vi "Chart_to_GraphXY.vi"(5 "Time window":u16=20, 6 "reference in":cluster{"Tempi":dbl[], "Valori":dbl[]}[](array[cluster])=[{"Tempi"=[], "Valori"=[]}], 7 "Function":T1, 8 "error in":errorcluster, 9 "Index plot":u8, 10 "Valore in":dbl=30.0, 11 "Tempo in":dbl) -> (0 "error out":errorcluster, 1 "Valori out":dbl[](array[numeric]), 2 "Tempo out":dbl[](array[numeric]), 3 "XY Graph":cluster{"Tempi":dbl[], "Valori":dbl[]}[](graph), 4 "reference out":cluster{"Tempi":dbl[], "Valori":dbl[]}[](array[cluster]))   [LabVIEW 2015, in "My Graphs.lvlib"]
uses:
  My Graphs.lvlib
  Chart to Graph enum.ctl
  <vilib>/Utility/error.llb/Error Cluster From Error Code.vi
  <vilib>/ErrorRing/Error Ring.xnode
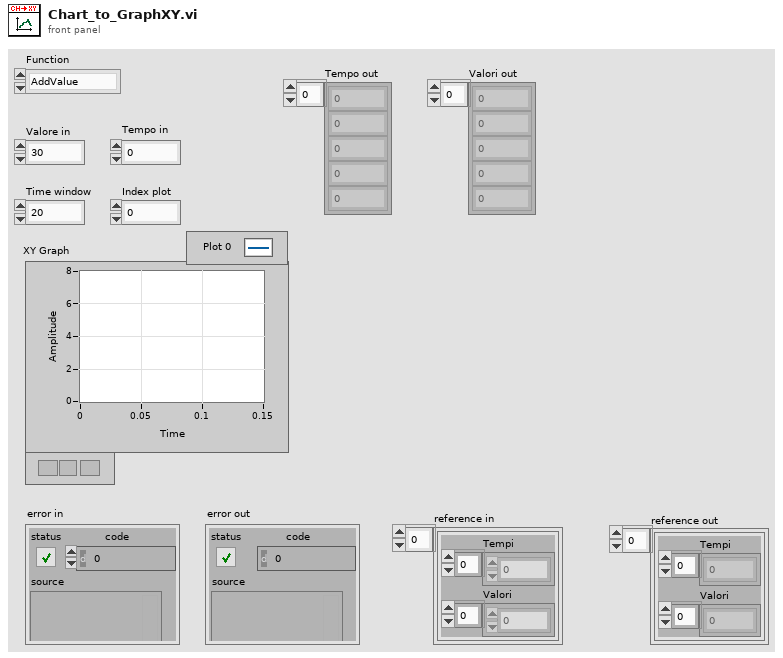
[diagram p1: front panel]
types:
  T1 = typedef "My Graphs.lvlib/Chart to Graph enum.ctl" = enum16{"AddValue", "Reset", "Delete_old"}
  T2 = cluster{"status":bool, "code":bool, "source":bool}
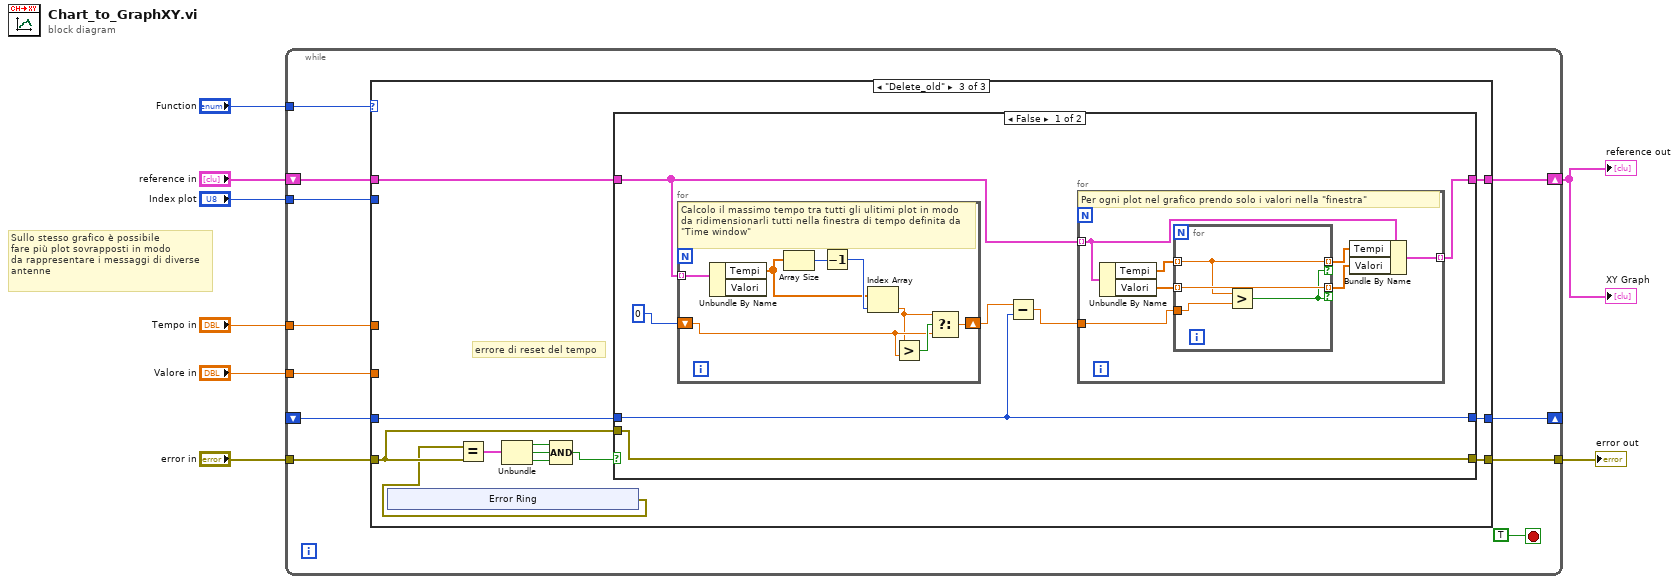
[diagram p0: block diagram]
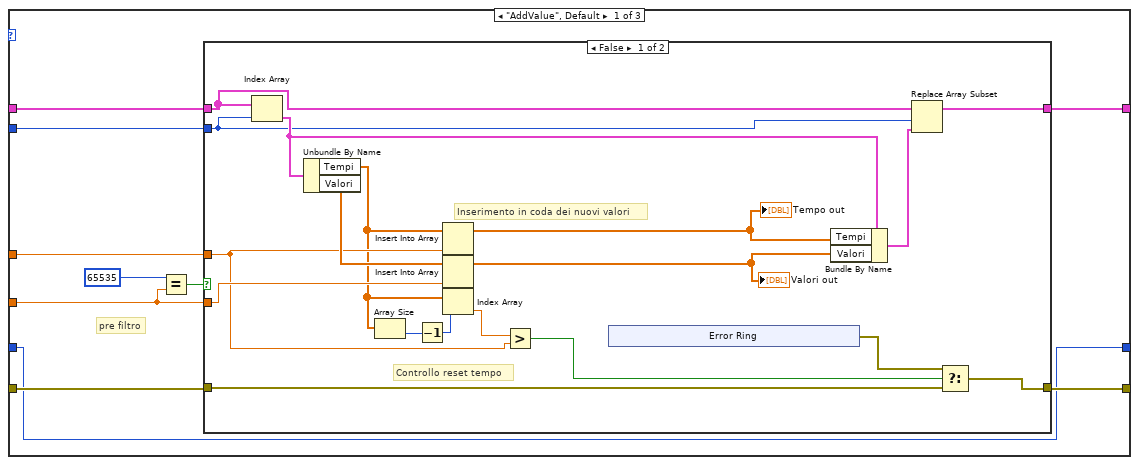
[diagram p2: hidden frame]
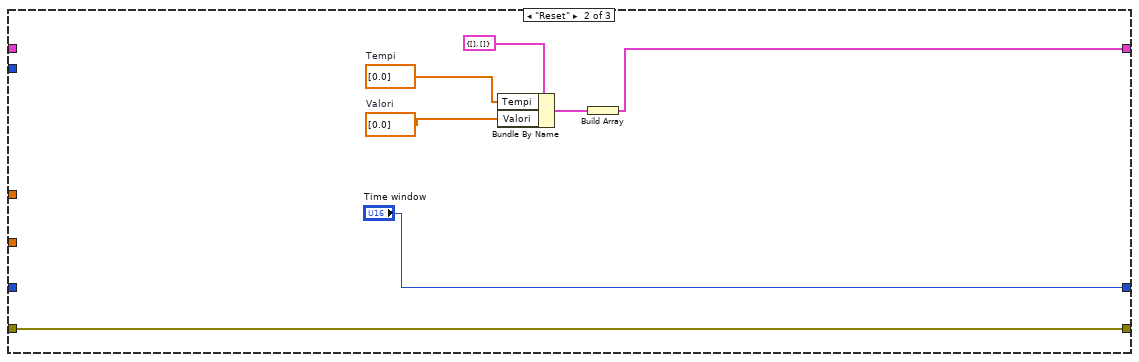
[diagram p4: hidden frame]
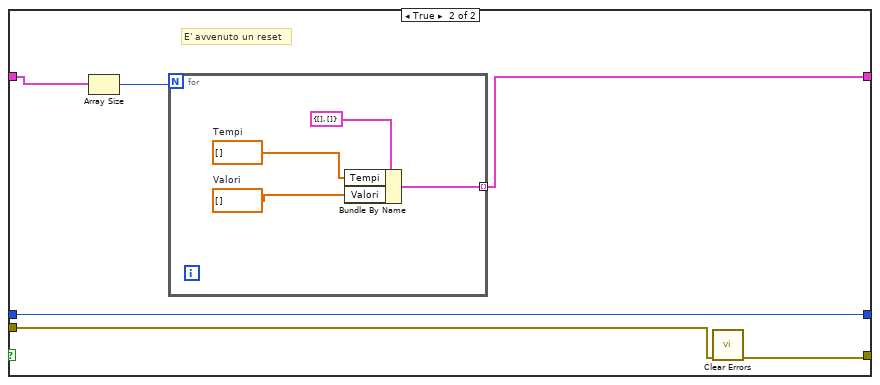
[diagram p5: hidden frame]
diagram:
  # "Sullo stesso grafico è possibile\nfare più plot sovrapposti in modo\nda rappresentare i messaggi di diverse\nantenne"
  n1 = while {
    tunnel: "Function" -> [w18]
    tunnel: "Tempo in" -> [w15]
    tunnel: "Valore in" -> [w12]
    tunnel: "error in" -> [w14]
    tunnel: [w13] -> w4
    tunnel: "Index plot" -> [w11]
    shift-right: [w17] -> w2
    shift-left: "reference in" -> [w16]
    shift-right: [w9] -> _
    shift-left: _ -> [w10]
    stop <- TRUE stop-if-true
    n2 = case shown="\"Delete_old\"" w18 {
      tunnel: w16 -> [w27 _ w73]
      tunnel: w15 -> [w29 _ _]
      tunnel: w12 -> [w25 _ _]
      tunnel: w14 -> [w24 w59 w64]
      tunnel: [w23 w59 w65] -> w13
      tunnel: [w26 w57 w71] -> w17
      tunnel: w11 -> [w28 _ _]
      tunnel: w10 -> [w20 _ w72]
      tunnel: [w20 "Time window" w63] -> w9
      frame "AddValue", Default {
        # "pre filtro"
        n3 = Equal?(x=65535, y=w25) -> (x = y?=w22:bool)
        n4 = case shown="False" w22 {
          tunnel: w29 -> [w40 _]
          tunnel: w28 -> [w33 _]
          tunnel: w27 -> [w35 w53]
          tunnel: [w45 w53] -> w26
          tunnel: w25 -> [w46 _]
          tunnel: w24 -> [w38 w54]
          tunnel: [w36 w54] -> w23
          frame False {
            # "Inserimento in coda dei nuovi valori"
            # "Controllo reset tempo"
            n5 = Index Array(array=w35, index=w33) -> (element=w34:cluster{"Tempi":dbl[], "Valori":dbl[]})
            n6 = Unbundle By Name(w34) -> ("Tempi"=w39:dbl[], "Valori"=w42:dbl[])
            n7 = Array Size(array=w39) -> (size(s)=w43:i32)
            n8 = Decrement(x=w43) -> (x-1=w44:i32)
            n9 = Insert Into Array(array=w39, new element=w40) -> (w31:dbl[])  [unwired: 1 in]
            "Tempo out" <- w31
            n10 = Insert Into Array(array=w42, new element=w46) -> (w30:dbl[])  [unwired: 1 in]
            "Valori out" <- w30
            n11 = Index Array(array=w39, index=w44) -> (element=w41:dbl)
            n12 = Greater?(x=w41, y=w40) -> (0:w37:bool)
            n13 = xnode "Error Ring"() -> ("error out"=w32:errorcluster)
            n14 = Bundle By Name(cluster=w34, "Tempi"=w31, "Valori"=w30) -> (w47:cluster{"Tempi":dbl[], "Valori":dbl[]})
            n15 = Replace Array Subset(array=w35, new element=w47, index=w33) -> (w45:cluster{"Tempi":dbl[], "Valori":dbl[]}[])
            n16 = Select(t=w32, s=w37, f=w38) -> (s? t:f=w36:errorcluster)
          }
          frame True {
          }
        }
      }
      frame "Reset" {
        w60 = dbl[] [0.0]  # Valori
        w61 = dbl[] [0.0]  # Tempi
        n17 = Bundle By Name(cluster=cluster{"Tempi":dbl[], "Valori":dbl[]} {"Tempi"=[], "Valori"=[]} ("input cluster"), "Tempi"=w61, "Valori"=w60) -> (w56:cluster{"Tempi":dbl[], "Valori":dbl[]})
        n18 = Build Array(w56) -> (w57:cluster{"Tempi":dbl[], "Valori":dbl[]}[])
      }
      frame "Delete_old" {
        # "errore di reset del tempo"
        n19 = xnode "Error Ring"() -> ("error out"=w62:errorcluster)
        n20 = Equal?(x=w62, y=w64) -> (x = y?=w70:T2)
        n21 = Unbundle(w70) -> ("status"=w69:bool, "code"=w68:bool, "source"=w67:bool)
        n22 = Compound Arithmetic op=AND(w69, w68, w67) -> (w66:bool)
        n23 = case shown="False" w66 {
          tunnel: w73 -> [w84 w109]
          tunnel: w72 -> [w79 w105]
          tunnel: [w81 w108] -> w71
          tunnel: [w80 w107] -> w65
          tunnel: w64 -> [w80 w106]
          tunnel: [w79 w105] -> w63
          frame False {
            n24 = for {
              tunnel: w84 -> [w104] mode=indexing
              shift-right: [w100] -> w83
              shift-left: 0 -> [w98]
              # "Calcolo il massimo tempo tra tutti gli ulitimi plot in modo da ridimensionarli tutti nella finestra di tempo definita da \"Time window\""
              n25 = Unbundle By Name(w104) -> ("Tempi"=w101:dbl[])  [unwired: 1 out]
              n26 = Array Size(array=w101) -> (size(s)=w103:i32)
              n27 = Decrement(x=w103) -> (x-1=w102:i32)
              n28 = Index Array(array=w101, index=w102) -> (element=w97:dbl)
              n29 = Greater?(x=w97, y=w98) -> (0:w99:bool)
              n30 = Select(t=w97, s=w99, f=w98) -> (s? t:f=w100:dbl)
            }
            n31 = Subtract(x=w83, y=w79) -> (x-y=w82:dbl)
            n32 = for {
              tunnel: w84 -> [w89] mode=indexing
              tunnel: w82 -> [w90]
              tunnel: [w86] -> w81 mode=indexing
              # "Per ogni plot nel grafico prendo solo i valori nella \"finestra\""
              n33 = Unbundle By Name(w89) -> ("Tempi"=w92:dbl[], "Valori"=w91:dbl[])
              n34 = for {
                tunnel: w92 -> [w94] mode=indexing
                tunnel: w91 -> [w96] mode=indexing
                tunnel: w90 -> [w95]
                tunnel: [w94] -> w88 mode=indexing if=w93
                tunnel: [w96] -> w87 mode=indexing if=w93
                n35 = Greater?(x=w94, y=w95) -> (0:w93:bool)
              }
              n36 = Bundle By Name(cluster=w89, "Tempi"=w88, "Valori"=w87) -> (w86:cluster{"Tempi":dbl[], "Valori":dbl[]})
            }
          }
          frame True {
            # "E' avvenuto un reset"
            n37 = Array Size(array=w109) -> (size(s)=w110:i32)
            n38 = for {
              N: w110 -> [_]
              tunnel: [w111] -> w108 mode=indexing
              w113 = dbl[] []  # Valori
              w114 = dbl[] []  # Tempi
              n39 = Bundle By Name(cluster=cluster{"Tempi":dbl[], "Valori":dbl[]} {"Tempi"=[], "Valori"=[]} ("input cluster"), "Tempi"=w114, "Valori"=w113) -> (w111:cluster{"Tempi":dbl[], "Valori":dbl[]})
            }
            n40 = call <vilib>:"Clear Errors.vi"("error in (no error)"=w106) -> ("error out"=w107:errorcluster)  [unwired: 5 in, 1 out]
          }
        }
      }
    }
  }
  "XY Graph" <- w2
  "error out" <- w4
  "reference out" <- w2
